vi "Text Description.vi"(11 "CancelableObserver in":refnum<class "CancelableObserver.lvclass">) -> (2 "Description":string, 3 "CancelableObserver out":refnum<class "CancelableObserver.lvclass">)   [LabVIEW 2011, in "Messenging.lvlib" / "CancelableObserver.lvclass"]
uses:
  CancelableObserver.lvclass
  SendOnly/Observer.lvclass
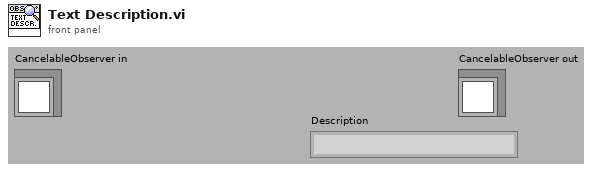
[diagram p1: front panel]
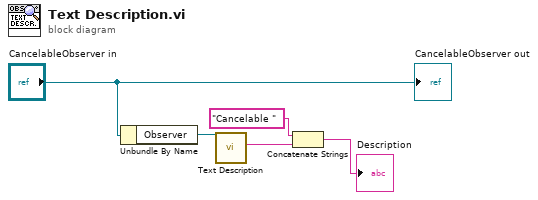
[diagram p0: block diagram]
diagram:
  n1 = Unbundle By Name("CancelableObserver in") -> ("Observer"=w5:refnum<class "Observer.lvclass">)
  n2 = call-dynamic "Text Description.vi"("Send in"=w5) -> ("Description"=w2:string)  [unwired: 10 out]
  n3 = Concatenate Strings("Cancelable " ("string"), w2) -> (→"Description":string)
  "CancelableObserver out" <- "CancelableObserver in"
